vi "Control.vi"() -> ()   [LabVIEW 2012]
uses:
  TryFunction.dll
panel:
  out "Numeric 2":dbl
  out "Numeric":dbl
  in  "Send Picture":bool
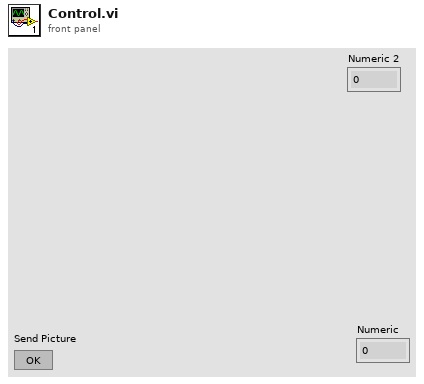
[diagram p1: front panel]
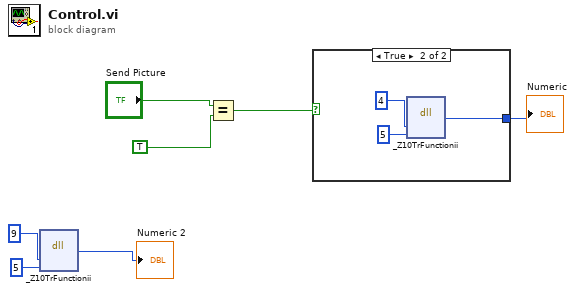
[diagram p0: block diagram]
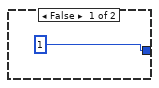
[diagram p2: hidden frame]
diagram:
  n1 = dll-call lib="C:/Users/abhinav/Documents/OMC/TryFunction.dll" fn="_Z10TrFunctionii"("a"=9, "b"=5) -> ("return type"=→"Numeric 2":i32)  [unwired: 5 in, 2 out]
  n2 = Equal?(x="Send Picture", y=TRUE) -> (x = y?=w5:bool)
  n3 = case shown="True" w5 {
    tunnel: [1 w9] -> w4
    frame False {
    }
    frame True {
      n4 = dll-call lib="C:/Users/abhinav/Documents/OMC/TryFunction.dll" fn="_Z10TrFunctionii"("a"=4, "b"=5) -> ("return type"=w9:i32)  [unwired: 5 in, 2 out]
    }
  }
  "Numeric" <- w4
